vi "Raw Protobuf.vi"() -> ()   [LabVIEW 2020]
uses:
  Source/Protobuf RAW/Helpers/Wire Chunk.ctl
  Source/Protobuf RAW/Type Serializer/Wire Type.ctl
  Source/Protobuf RAW/Message/Raw Message.lvclass
  E:/Labview/LV 2020/Libs/LV Protobuf Raw/Source/Protobuf RAW/Tag/Basic Type.lvclass
  Source/Protobuf RAW/sint32/sint32.lvclass/sint32.ctl
  Source/Protobuf RAW/uint32/uint32.lvclass/uint32.ctl
  Source/Protobuf RAW/string/string.lvclass/string.ctl
  Source/Protobuf RAW/float/float.lvclass/float.ctl
  Source/Protobuf RAW/packed/packed.lvclass/packed.ctl
  Source/Protobuf RAW/Message/Raw Message.lvclass/Raw Message.ctl
  Source/Protobuf RAW/float/Write Value.vi
  Source/Protobuf RAW/packed/Write Value.vi
  Source/Protobuf RAW/string/Write Value.vi
  Source/Protobuf RAW/uint32/Write Value.vi
  Source/Protobuf RAW/sint32/Write Value.vi
  Source/Protobuf RAW/Message/Read Tags.vi
  Source/Protobuf RAW/sint32/sint32.lvclass
  Source/Protobuf RAW/string/string.lvclass
  Source/Protobuf RAW/float/float.lvclass
  E:/Labview/LV 2020/Libs/LV Protobuf Raw/Source/Protobuf RAW/Scalar Encoder/Scalar Type.lvclass
  Source/Protobuf RAW/packed/packed.lvclass
  Source/Protobuf RAW/uint32/uint32.lvclass
  Source/Protobuf RAW/Scalar Encoder/Scalar Type.lvclass
  Source/Protobuf RAW/Tag/Basic Type.lvclass
  Source/Protobuf RAW.lvlib
  E:/Labview/LV 2020/Libs/LV Protobuf Raw/Source/Protobuf RAW/Proto Value/Proto Type.lvclass
  E:/Labview/LV 2020/Libs/LV Protobuf Raw/Source/Protobuf RAW/Type Serializer/Type Serializer.lvclass
  E:/Labview/LV 2020/Libs/LV Protobuf Raw/Source/Protobuf RAW/String Representable/String Representable.lvclass
  E:/Labview/LV 2020/Libs/LV Protobuf Raw/Source/Protobuf RAW/Wire Type Group/Wire Type Group.lvclass
  E:/Labview/LV 2020/Libs/LV Protobuf Raw/Source/Protobuf RAW/I32 Encoder/I32.lvclass
  E:/Labview/LV 2020/Libs/LV Protobuf Raw/Source/Protobuf RAW/float/float.lvclass
  Source/Protobuf RAW/Wire Type Group/Wire Type Group.lvclass
panel:
  out "Packed Floats":sgl[](array[numeric])
  out "Array":variant[](array[variant])
  in  "Tree":string(tree)
  out "String Representation":string
  out "String Representation Anonymous":string
  out "Value 2":i32
  out "Value":u32
  out "String Representation Deserialized":string
  out "Raw Fields":T1[](array[typedef])
  out "Message HEX":string
  out "Buffer":u8[](array[numeric]) format="%08b"
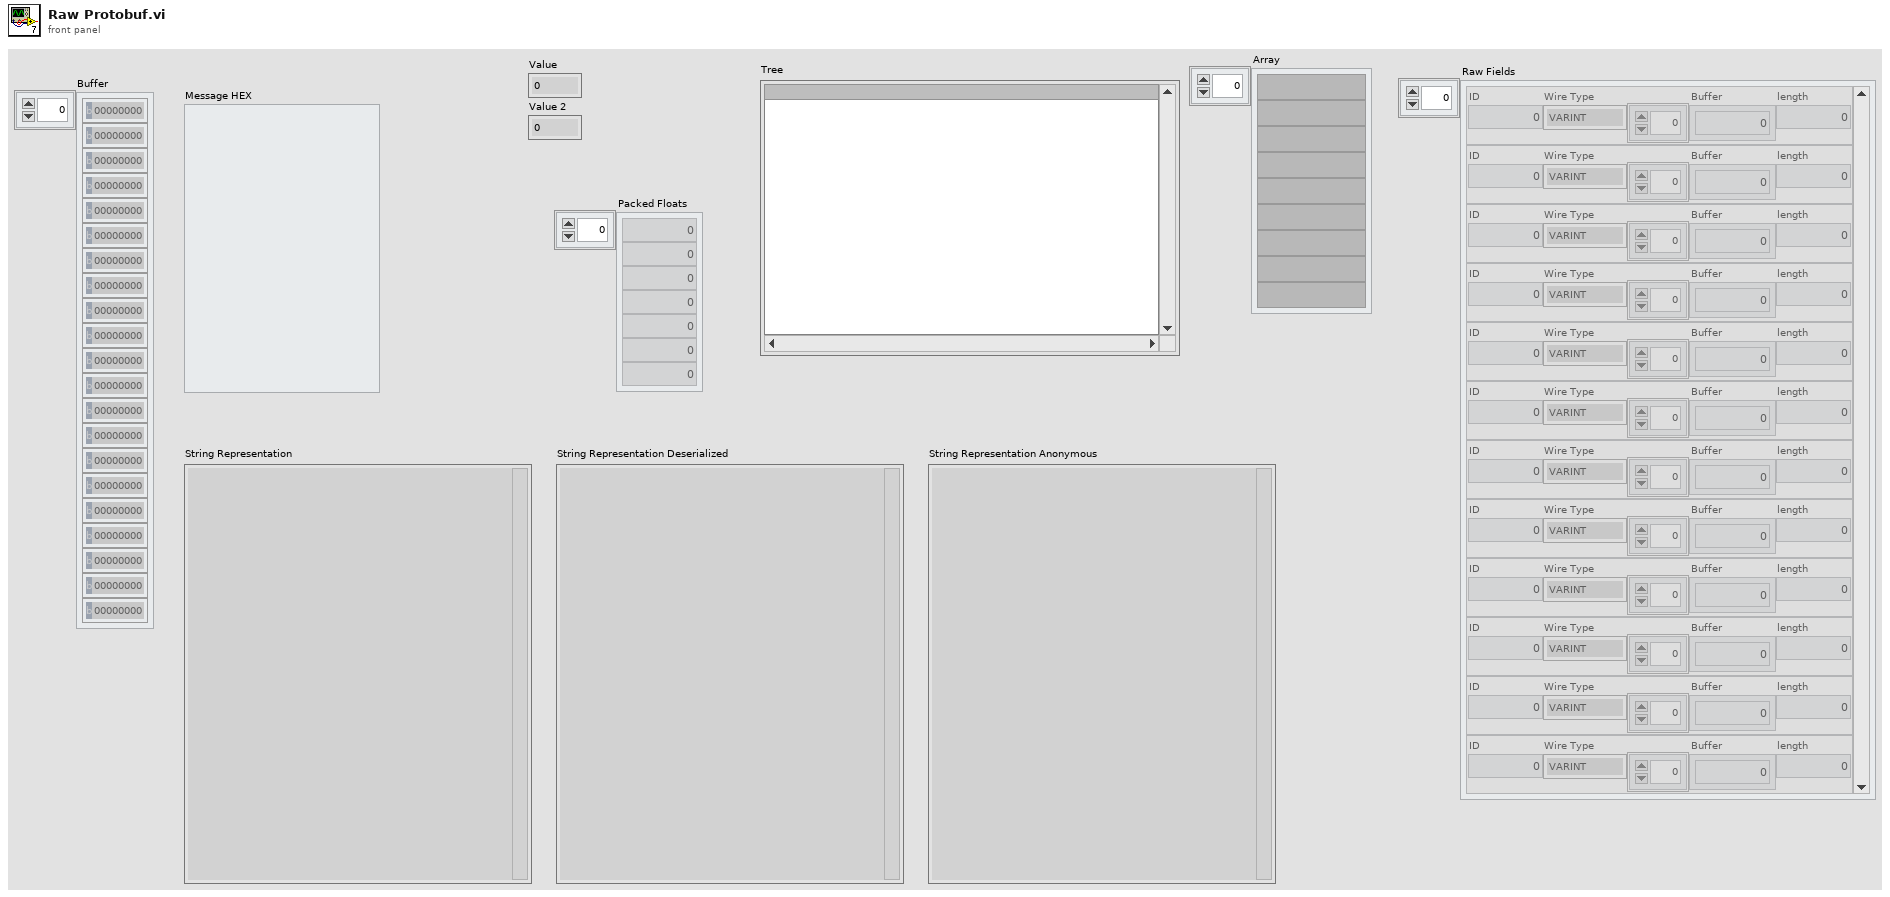
[diagram p1: front panel]
types:
  T1 = typedef "Protobuf RAW.lvlib/Wire Chunk.ctl" = cluster{"ID":u32, "Wire Type":T2, "Buffer":u8[], "length":i32}
  T2 = typedef "Protobuf RAW.lvlib/Wire Type Group.lvclass/Wire Type.ctl" = enum16{"VARINT", "I64", "LEN", "SGROUP", "EGROUP", "I32"}
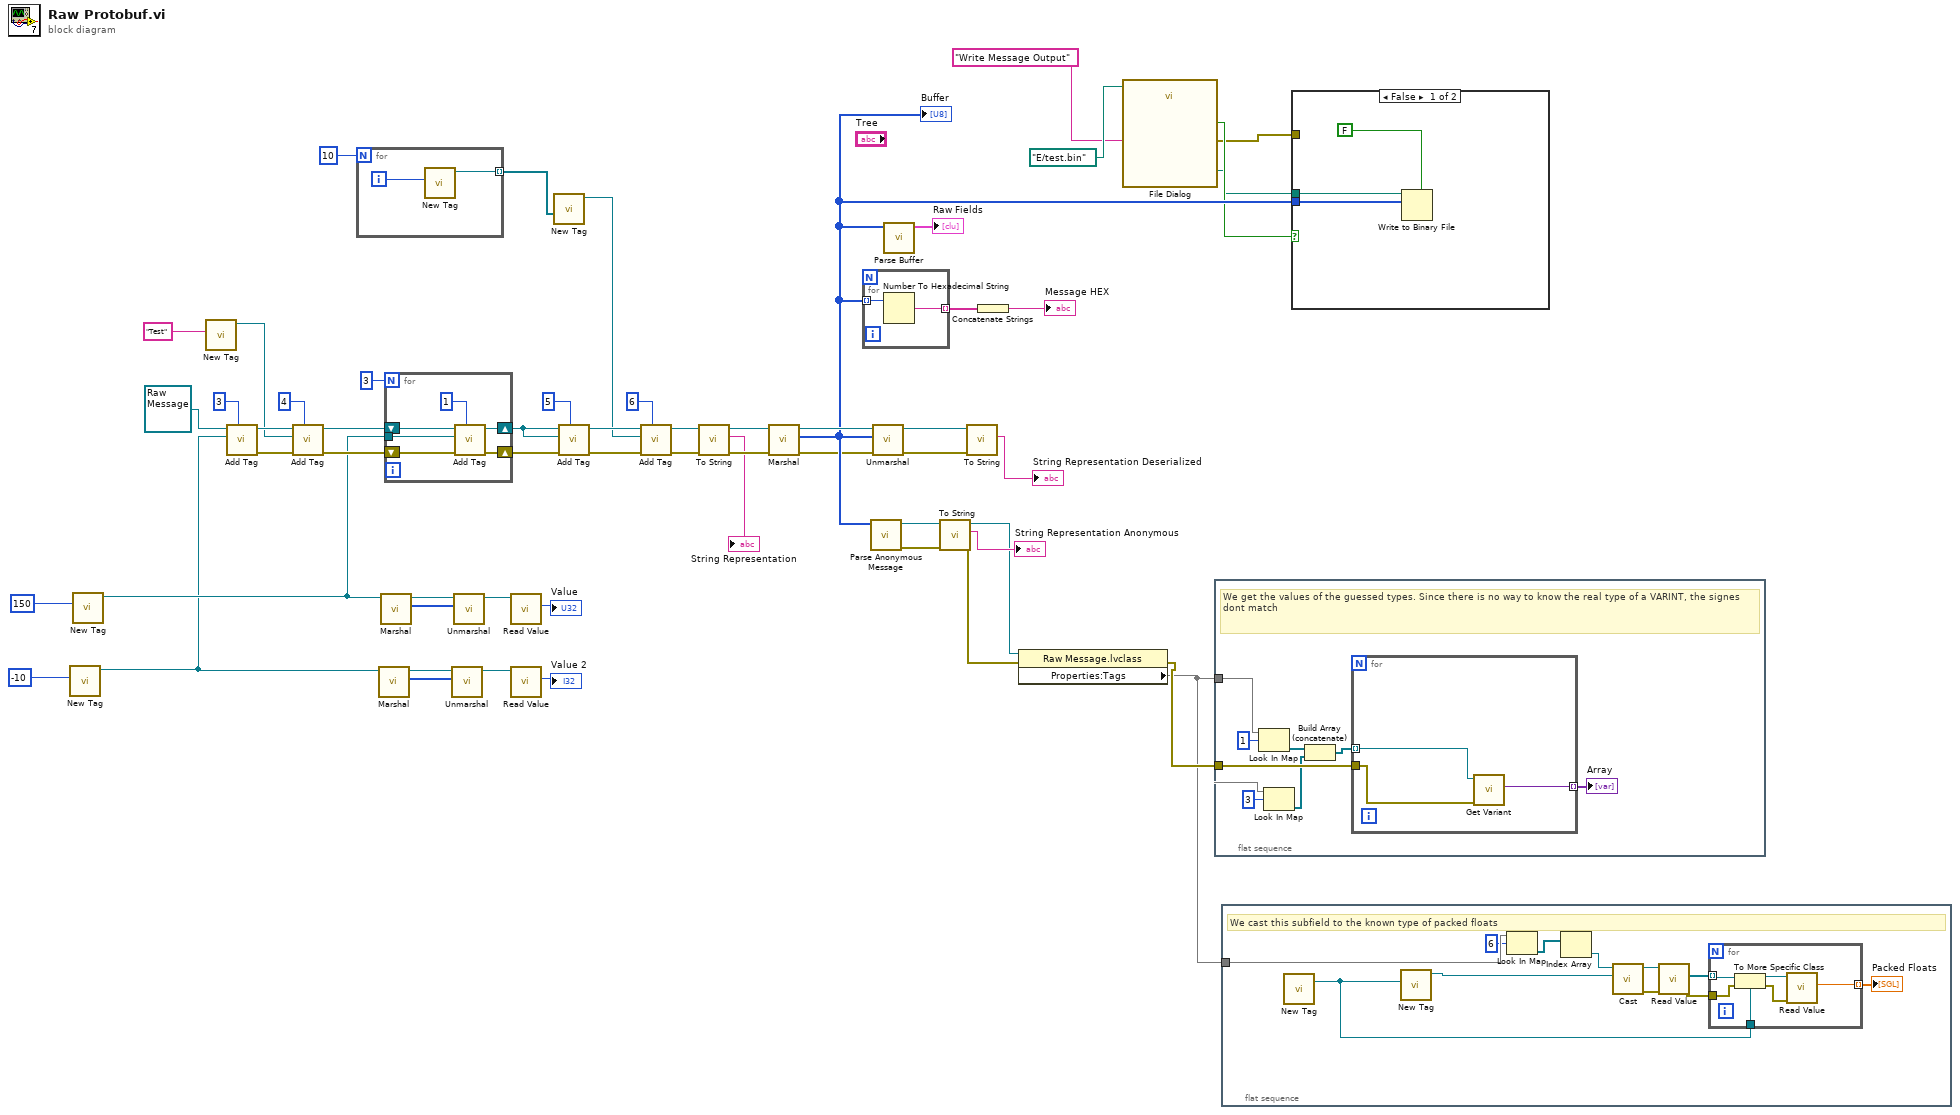
[diagram p0: block diagram]
diagram:
  n1 = call-poly "New Tag.vi"("Value"=-10) -> ("int32 out"=w24:refnum<class "sint32.lvclass">)  [unwired: 9 in, 1 out]
  n2 = call-poly "New Tag.vi"("Value"=u32 150) -> ("int32 out"=w30:refnum<class "uint32.lvclass">)  [unwired: 9 in, 1 out]
  n3 = call-poly "New Tag.vi"("Value"="Test") -> ("fixed32 out"=w43:refnum<class "string.lvclass">)  [unwired: 9 in, 1 out]
  n4 = call-dynamic "Add Tag.vi"("ID"=u32 3, "Tag Value"=w24, "Message in"=refnum<class "Raw Message.lvclass"> refnum ("Message.lvclass")) -> ("error out"=w56:errorcluster, "Message out"=w45:refnum<class "Raw Message.lvclass">)  [unwired: 7 in]
  n5 = call-dynamic "Add Tag.vi"("ID"=u32 4, "error in (no error)"=w56, "Tag Value"=w43, "Message in"=w45) -> ("error out"=w46:errorcluster, "Message out"=w44:refnum<class "Raw Message.lvclass">)  [unwired: 6 in]
  n6 = for {
    N: 10 -> [_]
    tunnel: [w58] -> w16 mode=indexing
    i -> [w59]
    n7 = call-poly "New Tag.vi"("Value"=w59) -> ("float out"=w58:refnum<class "float.lvclass">)  [unwired: 9 in, 1 out]
  }
  n8 = call-dynamic "Marshal.vi"("int32 in"=w24) -> ("Buffer"=w26:u8[], "int32 out"=w25:refnum<class "sint32.lvclass">)  [unwired: 8 in, 1 out]
  n9 = call-dynamic "Marshal.vi"("int32 in"=w30) -> ("Buffer"=w29:u8[], "int32 out"=w31:refnum<class "uint32.lvclass">)  [unwired: 8 in, 1 out]
  n10 = for {
    N: 3 -> [_]
    tunnel: w30 -> [w61]
    shift-right: [w64] -> w52
    shift-left: w46 -> [w65]
    shift-right: [w62] -> w39
    shift-left: w44 -> [w63]
    n11 = call-dynamic "Add Tag.vi"("ID"=u32 1, "error in (no error)"=w65, "Tag Value"=w61, "Message in"=w63) -> ("error out"=w64:errorcluster, "Message out"=w62:refnum<class "Raw Message.lvclass">)  [unwired: 6 in]
  }
  n12 = call-dynamic "Unmarshal.vi"("Buffer"=w26, "int32 in"=w25) -> ("int32 out"=w23:refnum<class "sint32.lvclass">)  [unwired: 7 in, 2 out]
  n13 = call-dynamic "Unmarshal.vi"("Buffer"=w29, "int32 in"=w31) -> ("int32 out"=w28:refnum<class "uint32.lvclass">)  [unwired: 7 in, 2 out]
  n14 = call "Read Value.vi"("int32 in"=w28) -> ("Value"=→"Value":u32)  [unwired: 8 in, 2 out]
  n15 = call "Read Value.vi"("int32 in"=w23) -> ("Value"=→"Value 2":i32)  [unwired: 8 in, 2 out]
  n16 = call-poly "New Tag.vi"("Value"=w16) -> ("fixed32 out"=w34:refnum<class "packed.lvclass">)  [unwired: 9 in, 1 out]
  n17 = call-dynamic "Add Tag.vi"("ID"=u32 5, "error in (no error)"=w52, "Tag Value"=w39, "Message in"=w39) -> ("error out"=w40:errorcluster, "Message out"=w36:refnum<class "Raw Message.lvclass">)  [unwired: 6 in]
  n18 = call-dynamic "Add Tag.vi"("ID"=u32 6, "error in (no error)"=w40, "Tag Value"=w34, "Message in"=w36) -> ("error out"=w12:errorcluster, "Message out"=w14:refnum<class "Raw Message.lvclass">)  [unwired: 6 in]
  n19 = call-dynamic "To String.vi"("error in (no error)"=w12, "Raw Message in"=w14) -> ("error out"=w11:errorcluster, "String Representation"=→"String Representation":string, "Raw Message out"=w13:refnum<class "Raw Message.lvclass">)  [unwired: 7 in]
  n20 = call-dynamic "Marshal.vi"("error in (no error)"=w11, "Message in"=w13) -> ("error out"=w20:errorcluster, "Buffer"=w21:u8[], "Message out"=w54:refnum<class "Raw Message.lvclass">)  [unwired: 7 in]
  "Buffer" <- w21
  n21 = for {
    tunnel: w21 -> [w67] mode=indexing
    tunnel: [w66] -> w51 mode=indexing
    n22 = Number To Hexadecimal String(2:w67) -> (0:w66:string)  [unwired: 1 in]
  }
  n23 = call "Parse Anonymous Message.vi"("Buffer"=w21) -> ("error out"=w19:errorcluster, "Raw Message"=w18:refnum<class "Raw Message.lvclass">)  [unwired: 8 in, 1 out]
  n24 = call-dynamic "Unmarshal.vi"("error in (no error)"=w20, "Buffer"=w21, "Message in"=w54) -> ("error out"=w32:errorcluster, "Message out"=w53:refnum<class "Raw Message.lvclass">)  [unwired: 6 in, 1 out]
  n25 = call "Parse Buffer.vi"("Buffer"=w21) -> ("Raw Fields"=→"Raw Fields":T1[])  [unwired: 9 in, 1 out]
  n26 = call-dynamic "To String.vi"("error in (no error)"=w19, "Raw Message in"=w18) -> ("error out"=w8:errorcluster, "String Representation"=→"String Representation Anonymous":string, "Raw Message out"=w9:refnum<class "Raw Message.lvclass">)  [unwired: 7 in]
  n27 = call-dynamic "To String.vi"("error in (no error)"=w32, "Raw Message in"=w53) -> ("String Representation"=→"String Representation Deserialized":string)  [unwired: 7 in, 2 out]
  n28 = Concatenate Strings(w51) -> (→"Message HEX":string)
  n29 = property class="Raw Message.lvclass"(reference=w9, error in=w8) -> (error out=w7:errorcluster, "Properties:Tags"=w1:map{u32, refnum<class "Basic Type.lvclass">[]})  [unwired: 1 out]
  n30 = call "File Dialog"("start path"=path "E:/test.bin" ("file (use dialog)"), "prompt"="Write Message Output") -> ("selected path"=w3:path, "cancelled"=w5:bool, "error out"=w4:errorcluster)  [unwired: 10 in, 1 out]
  n31 = flat-sequence {
    tunnel: w7 -> [w73]
    tunnel: w1 -> [w68]
    frame #0 {
      # "We get the values of the guessed types. Since there is no way to know the real type of a VARINT, the signes dont match"
      n32 = Look In Map(map=w68, key=u32 1) -> (value=w74:refnum<class "Basic Type.lvclass">[])  [unwired: 1 in, 1 out]
      n33 = Look In Map(map=w68, key=u32 3) -> (value=w69:refnum<class "Basic Type.lvclass">[])  [unwired: 1 in, 1 out]
      n34 = Build Array (concatenate)(w74, w69) -> (w70:refnum<class "Basic Type.lvclass">[])
      n35 = for {
        tunnel: w70 -> [w76] mode=indexing
        tunnel: w73 -> [w78]
        tunnel: [w77] -> w72 mode=indexing
        n36 = call-dynamic "Get Variant.vi"("error in (no error)"=w78, "Type Serializer in"=w76) -> ("Variant"=w77:variant)  [unwired: 7 in, 2 out]
      }
      "Array" <- w72
    }
  }
  n37 = flat-sequence {
    tunnel: w1 -> [w89]
    frame #0 {
      # "We cast this subfield to the known type of packed floats"
      n38 = call-poly "New Tag.vi"() -> ("float out"=w82:refnum<class "float.lvclass">)  [unwired: 10 in, 1 out]
      n39 = call-poly "New Tag.vi"("Type"=w82) -> ("fixed32 out"=w87:refnum<class "packed.lvclass">)  [unwired: 9 in, 1 out]
      n40 = Look In Map(map=w89, key=u32 6) -> (value=w86:refnum<class "Basic Type.lvclass">[])  [unwired: 1 in, 1 out]
      n41 = Index Array(array=w86) -> (element=w85:refnum<class "Basic Type.lvclass">)  [unwired: 1 in]
      n42 = call "Cast.vi"("Cast Type"=w87, "Basic Type in"=w85) -> ("error out"=w83:errorcluster, "Basic Type out"=w84:refnum<class "packed.lvclass">)  [unwired: 8 in]
      n43 = call "Read Value.vi"("error in (no error)"=w83, "fixed32 in"=w84) -> ("error out"=w81:errorcluster, "Value"=w79:refnum<class "Scalar Type.lvclass">[])  [unwired: 7 in, 1 out]
      n44 = for {
        tunnel: w79 -> [w95] mode=indexing
        tunnel: w82 -> [w94]
        tunnel: w81 -> [w93]
        tunnel: [w90] -> w80 mode=indexing
        n45 = To More Specific Class(target class=w94, reference=w95, error in=w93) -> (specific class reference=w92:refnum<class "float.lvclass">, error out=w91:errorcluster)
        n46 = call "Read Value.vi"("error in (no error)"=w91, "float in"=w92) -> ("Value"=w90:sgl)  [unwired: 7 in, 2 out]
      }
      "Packed Floats" <- w80
    }
  }
  n47 = case shown="False" w5 {
    tunnel: w21 -> [w97 _]
    tunnel: w3 -> [w96 _]
    tunnel: w4 -> [_ _]
    frame False {
      n48 = Write to Binary File(file (use dialog)=w96, data=w97, 5:FALSE ("prepend array or string size? (T)")) -> ()  [unwired: 3 in, 3 out]
    }
    frame True {
    }
  }
